vi "WriteRefFromFile.vi"(8 "error in (no error)":errorcluster caption="entrée d'erreur (pas d'erreur)", 9 "Position Codeur En Pas":i32, 10 "Numéro de la référence":u16, 11 "Entrée Variables d'Axes":T1) -> (0 "error out":errorcluster caption="sortie d'erreur")   [LabVIEW 2013]
uses:
  Controls/AdressesVariablesPartagees.ctl
  <vilib>/regexp/Match Regular Expression.xnode
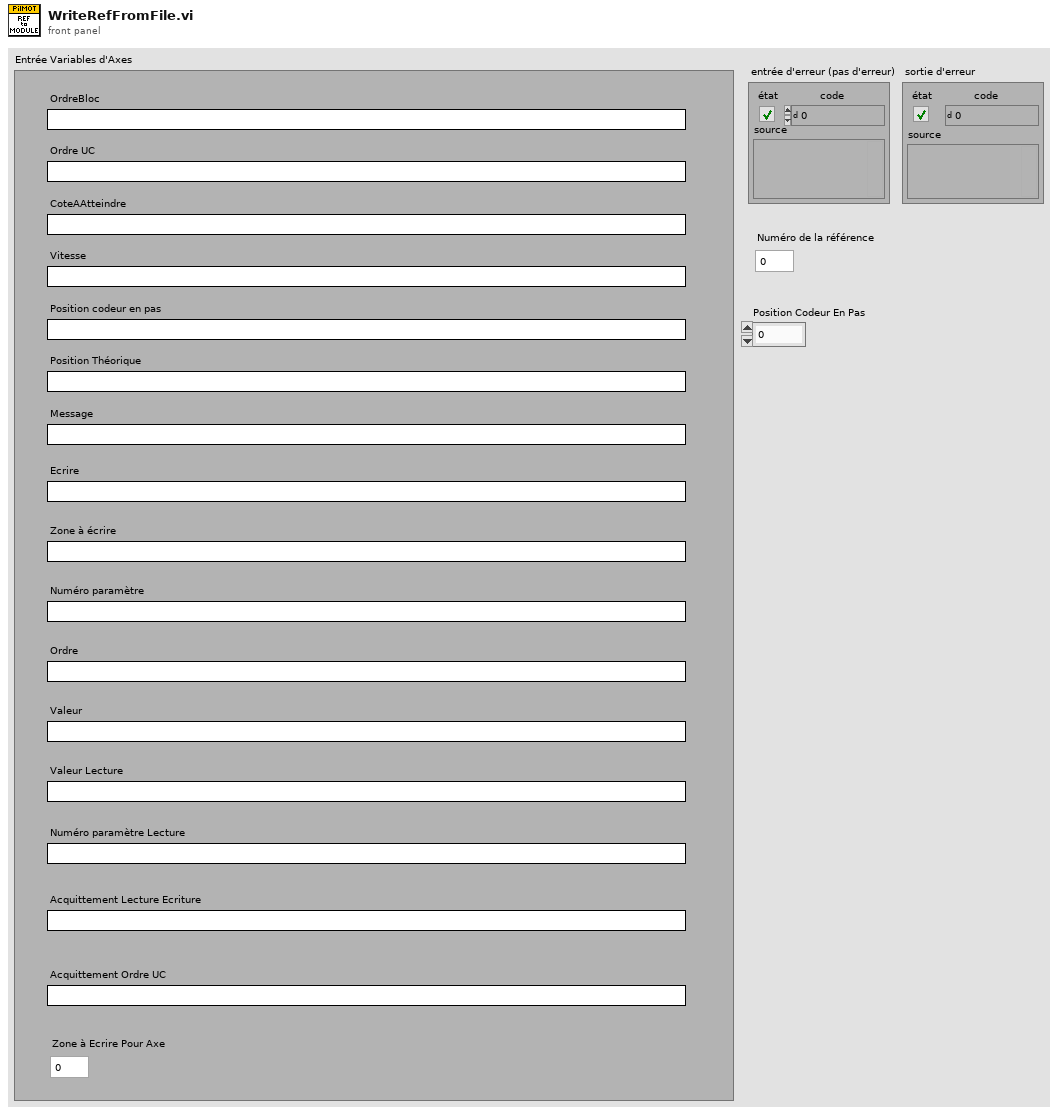
[diagram p1: front panel]
types:
  T1 = typedef "AdressesVariablesPartagees.ctl" = cluster{"OrdreBloc":string, "Ordre UC":string, "CoteAAtteindre":string, "Vitesse":string, "Position codeur en pas":string, "Position Théorique":string, "Message":string, "Ecrire":string, "Zone à écrire":string, "Numéro paramètre":string, "Ordre":string, "Valeur":string, "Valeur Lecture":string, "Numéro paramètre Lecture":string, "Acquittement Lecture Ecriture":string, "Zone à Ecrire Pour Axe ":u16, "Acquittement Ordre UC":string}
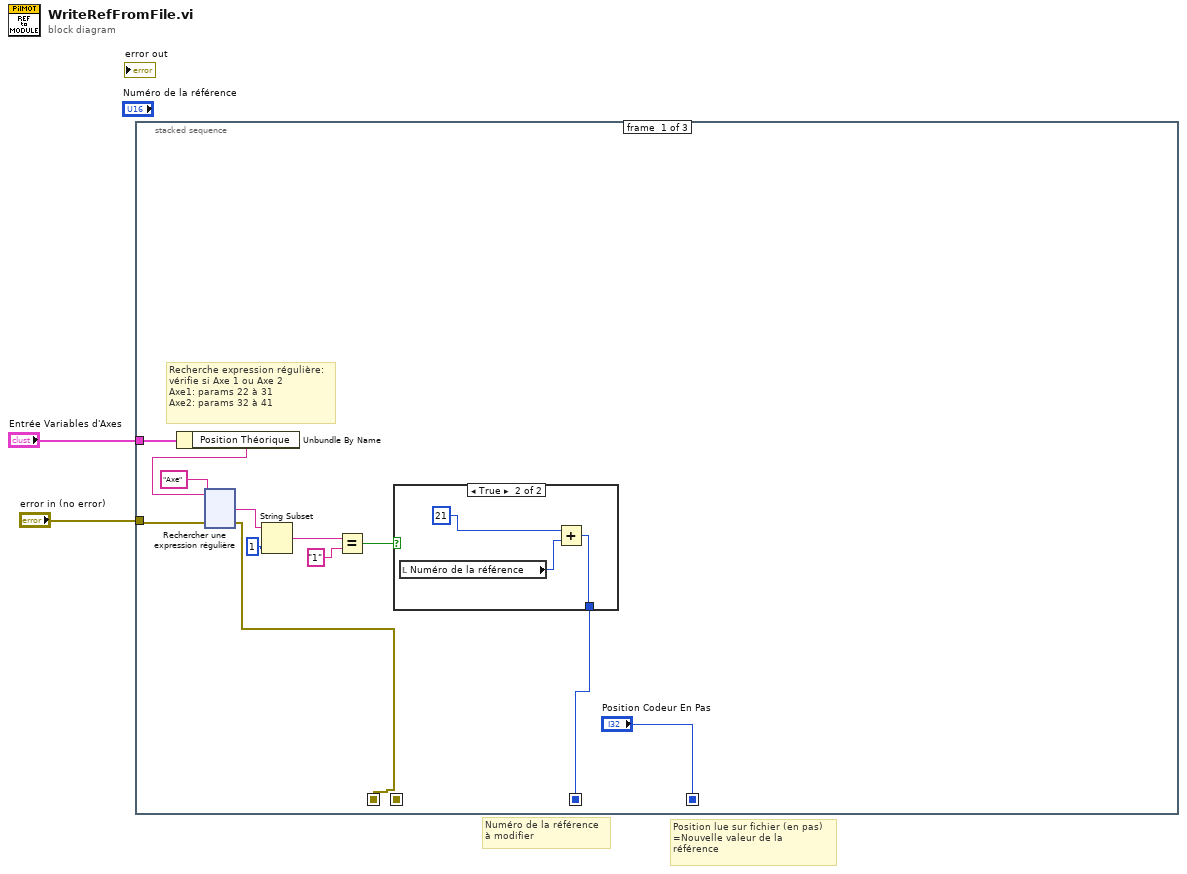
[diagram p0: block diagram]
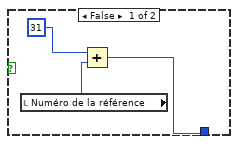
[diagram p2: hidden frame]
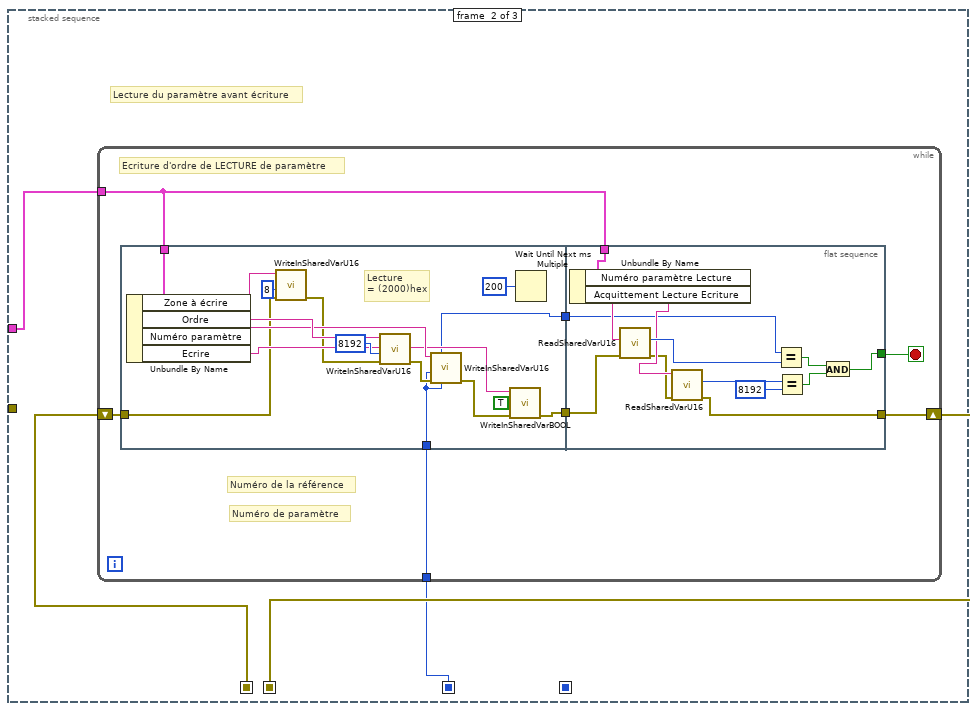
[diagram p3: hidden frame]
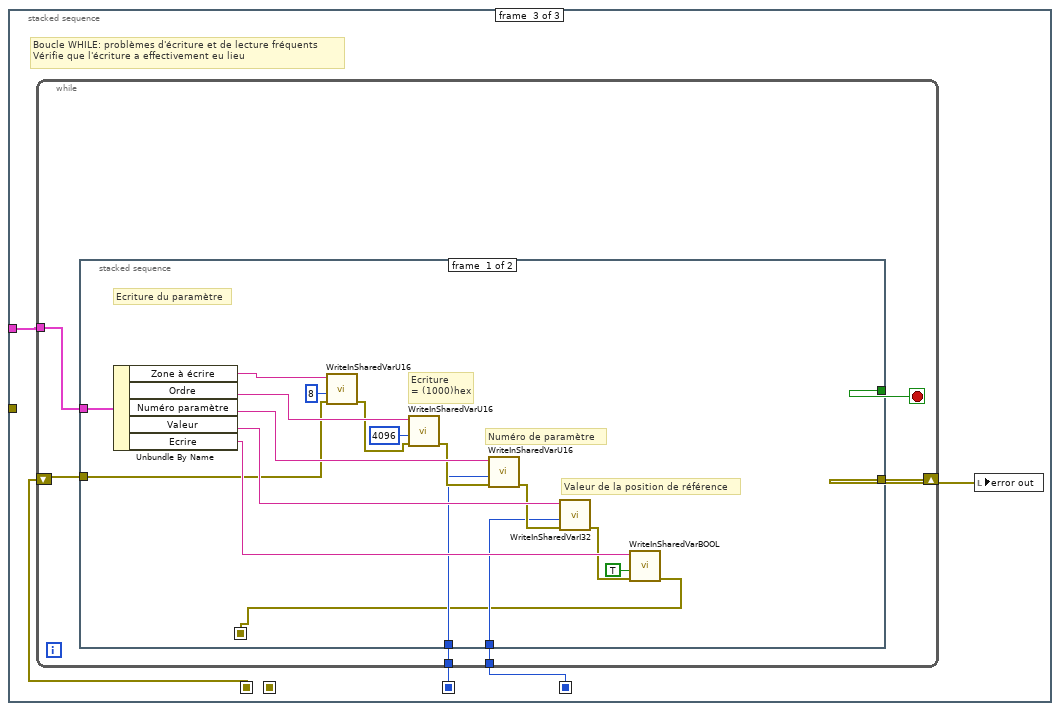
[diagram p4: hidden frame]
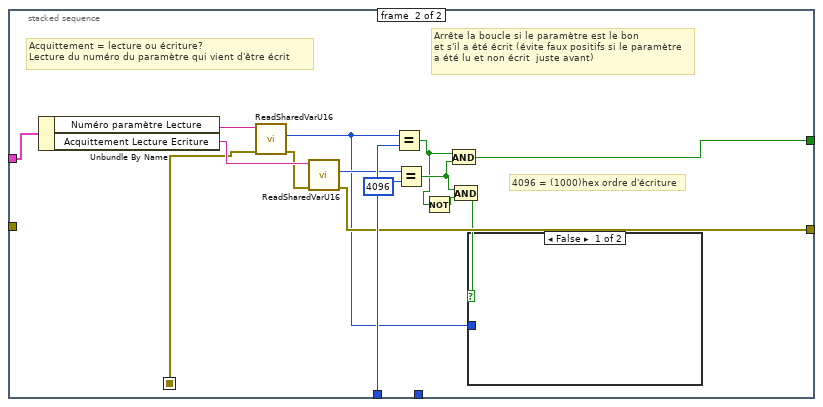
[diagram p5: hidden frame]
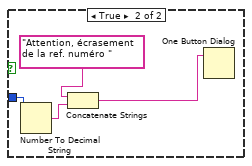
[diagram p6: hidden frame]
diagram:
  # "Position lue sur fichier (en pas)\n=Nouvelle valeur de la \nréférence"
  # "Numéro de la référence\nà modifier"
  n1 = stacked-sequence {
    seq-local: [w3 _ _] -> [_ w138 w175]
    seq-local: [w7 _ _] -> [_ w135 w177]
    seq-local: ["Position Codeur En Pas" _ _] -> [_ _ w176]
    seq-local: [_ w136 _] -> [_ _ _]
    tunnel: "Entrée Variables d'Axes" -> [w14 w137 w178]
    tunnel: "error in (no error)" -> [w6 _ _]
    frame #0 {
      # "Recherche expression régulière:\nvérifie si Axe 1 ou Axe 2\nAxe1: params 22 à 31\nAxe2: params 32 à 41"
      n2 = Unbundle By Name(w14) -> ("Position Théorique"=w5:string)
      n3 = xnode "Rechercher une expression régulière"("chaîne en entrée"=w5, "expression régulière"="Axe", "entrée d'erreur"=w6) -> ("après la correspondance"=w12:string, "sortie d'erreur"=w3:errorcluster)  [unwired: 3 in, 3 out]
      n4 = String Subset(string=w12, length (rest)=1 ("longueur (reste)")) -> (substring=w9:string)  [unwired: 1 in]
      n5 = Equal?(x=w9, y="1") -> (x = y?=w8:bool)
      n6 = case shown="True" w8 {
        tunnel: [w15 w18] -> w7
        frame False {
          n7 = local read "Numéro de la référence"() -> (w16:u16)
          n8 = Add(x=u16 31 ("Offset Paramètre"), y=w16) -> (x+y=w15:u16)
        }
        frame True {
          n9 = local read "Numéro de la référence"() -> (w19:u16)
          n10 = Add(x=u16 21 ("Offset Paramètre"), y=w19) -> (x+y=w18:u16)
        }
      }
    }
    frame #1 {
      # "Lecture du paramètre avant écriture"
      n11 = while {
        tunnel: w137 -> [w143]
        shift-right: [w142] -> w136
        shift-left: w138 -> [w141]
        tunnel: w135 -> [w139]
        stop <- w144 stop-if-true
        # "Numéro de la référence"
        # "Ecriture d'ordre de LECTURE de paramètre"
        # "Numéro de paramètre"
        n12 = flat-sequence {
          tunnel: w143 -> [w160]
          tunnel: [w153] -> w145
          tunnel: w141 -> [w148]
          tunnel: [w147] -> w140
          tunnel: w139 -> [w147]
          tunnel: [w165] -> w142
          tunnel: w145 -> [w171]
          tunnel: [w162] -> w144
          tunnel: w143 -> [w173]
          tunnel: w140 -> [w161]
          frame #0 {
            # "Lecture \n= (2000)hex"
            n13 = Unbundle By Name(w160) -> ("Zone à écrire"=w152:string, "Ordre"=w159:string, "Numéro paramètre"=w157:string, "Ecrire"=w155:string)
            n14 = call "WriteInSharedVarU16.vi"("entrée d'erreur (pas d'erreur)"=w148, "données en entrée"=u16 8, "refnum de variable partagée en entrée"=w152) -> ("sortie d'erreur"=w150:errorcluster)  [unwired: 8 in]
            n15 = call "WriteInSharedVarU16.vi"("entrée d'erreur (pas d'erreur)"=w150, "données en entrée"=u16 8192, "refnum de variable partagée en entrée"=w159) -> ("sortie d'erreur"=w156:errorcluster)  [unwired: 8 in]
            n16 = call "WriteInSharedVarU16.vi"("entrée d'erreur (pas d'erreur)"=w156, "données en entrée"=w147, "refnum de variable partagée en entrée"=w157) -> ("sortie d'erreur"=w154:errorcluster)  [unwired: 8 in]
            n17 = call "WriteInSharedVarBOOL.vi"("entrée d'erreur (pas d'erreur)"=w154, "données en entrée"=TRUE, "refnum de variable partagée en entrée"=w155) -> ("sortie d'erreur"=w153:errorcluster)  [unwired: 8 in]
            n18 = Wait Until Next ms Multiple(millisecond multiple=u32 200 ("n millisecondes")) -> ()  [unwired: 1 out]
          }
          frame #1 {
            n19 = Unbundle By Name(w173) -> ("Numéro paramètre Lecture"=w172:string, "Acquittement Lecture Ecriture"=w169:string)
            n20 = call "ReadSharedVarU16.vi"("entrée d'erreur (pas d'erreur)"=w171, "refnum de variable partagée en entrée"=w172) -> ("sortie d'erreur"=w166:errorcluster, "données en sortie"=w170:u16)  [unwired: 8 in]
            n21 = call "ReadSharedVarU16.vi"("entrée d'erreur (pas d'erreur)"=w166, "refnum de variable partagée en entrée"=w169) -> ("sortie d'erreur"=w165:errorcluster, "données en sortie"=w168:u16)  [unwired: 8 in]
            n22 = Equal?(x=w161, y=w170) -> (x = y?=w164:bool)
            n23 = Equal?(x=w168, y=u16 8192) -> (x = y?=w163:bool)
            n24 = And(x=w164, y=w163) -> (x .and. y?=w162:bool)
          }
        }
      }
    }
    frame #2 {
      # "Boucle WHILE: problèmes d'écriture et de lecture fréquents\nVérifie que l'écriture a effectivement eu lieu"
      n25 = while {
        tunnel: w178 -> [w184]
        tunnel: w177 -> [w183]
        tunnel: w176 -> [w182]
        shift-right: [w179] -> w174
        shift-left: w175 -> [w181]
        stop <- w180 stop-if-true
        n26 = stacked-sequence {
          seq-local: [w185 _] -> [_ w202]
          tunnel: w184 -> [w201 w216]
          tunnel: w183 -> [w189 w214]
          tunnel: w182 -> [w188 _]
          tunnel: w181 -> [w186 _]
          tunnel: [_ w209] -> w180
          tunnel: [_ w208] -> w179
          frame #0 {
            # "Ecriture du paramètre"
            # "Valeur de la position de référence"
            # "Numéro de paramètre"
            # "Ecriture \n= (1000)hex"
            n27 = Unbundle By Name(w201) -> ("Zone à écrire"=w200:string, "Ordre"=w198:string, "Numéro paramètre"=w196:string, "Valeur"=w195:string, "Ecrire"=w194:string)
            n28 = call "WriteInSharedVarU16.vi"("entrée d'erreur (pas d'erreur)"=w186, "données en entrée"=u16 8, "refnum de variable partagée en entrée"=w200) -> ("sortie d'erreur"=w193:errorcluster)  [unwired: 8 in]
            n29 = call "WriteInSharedVarU16.vi"("entrée d'erreur (pas d'erreur)"=w193, "données en entrée"=u16 4096, "refnum de variable partagée en entrée"=w198) -> ("sortie d'erreur"=w192:errorcluster)  [unwired: 8 in]
            n30 = call "WriteInSharedVarU16.vi"("entrée d'erreur (pas d'erreur)"=w192, "données en entrée"=w189, "refnum de variable partagée en entrée"=w196) -> ("sortie d'erreur"=w191:errorcluster)  [unwired: 8 in]
            n31 = call "WriteInSharedVarI32.vi"("entrée d'erreur (pas d'erreur)"=w191, "données en entrée"=w188, "refnum de variable partagée en entrée"=w195) -> ("sortie d'erreur"=w190:errorcluster)  [unwired: 8 in]
            n32 = call "WriteInSharedVarBOOL.vi"("entrée d'erreur (pas d'erreur)"=w190, "données en entrée"=TRUE, "refnum de variable partagée en entrée"=w194) -> ("sortie d'erreur"=w185:errorcluster)  [unwired: 8 in]
          }
          frame #1 {
            # "4096 = (1000)hex ordre d'écriture"
            # "Arrête la boucle si le paramètre est le bon\net s'il a été écrit (évite faux positifs si le paramètre\na été lu et non écrit  juste avant)"
            # "Acquittement = lecture ou écriture? \nLecture du numéro du paramètre qui vient d'être écrit"
            n33 = Unbundle By Name(w216) -> ("Numéro paramètre Lecture"=w215:string, "Acquittement Lecture Ecriture"=w213:string)
            n34 = call "ReadSharedVarU16.vi"("entrée d'erreur (pas d'erreur)"=w202, "refnum de variable partagée en entrée"=w215) -> ("sortie d'erreur"=w212:errorcluster, "données en sortie"=w203:u16)  [unwired: 8 in]
            n35 = call "ReadSharedVarU16.vi"("entrée d'erreur (pas d'erreur)"=w212, "refnum de variable partagée en entrée"=w213) -> ("sortie d'erreur"=w208:errorcluster, "données en sortie"=w211:u16)  [unwired: 8 in]
            n36 = Equal?(x=w203, y=w214) -> (x = y?=w205:bool)
            n37 = Equal?(x=w211, y=u16 4096) -> (x = y?=w207:bool)
            n38 = Not(x=w205) -> (.not. x?=w206:bool)
            n39 = And(x=w205, y=w207) -> (x .and. y?=w209:bool)
            n40 = And(x=w207, y=w206) -> (x .and. y?=w204:bool)
            n41 = case shown="False" w204 {
              tunnel: w203 -> [_ w220]
              frame False {
              }
              frame True {
                n42 = Number To Decimal String(number=w220) -> (decimal integer string=w219:string)  [unwired: 1 in]
                n43 = Concatenate Strings("Attention, écrasement de la ref. numéro " ("message"), w219) -> (w217:string)
                n44 = One Button Dialog(message=w217) -> ()  [unwired: 1 in, 1 out]
              }
            }
          }
        }
      }
      n45 = local write "error out"(w174) -> ()
    }
  }
